vi "integer to 7-seg decoder_special.vi"(0 "Integer number":u16, 2 "Display On/Off":bool, 5 "Is negative? (F)":bool) -> (7 "7-seg digit for negative":T1)   [LabVIEW 2015]
doc: "This module is intended only to display a possible error condition 'E', entering the number 8, and turn on the g segment to indicate a minus sign. Finally, it has a complete shutdown of the display, and this state takes precedence over all others."
uses:
  controls/green 7-seg display special.ctl
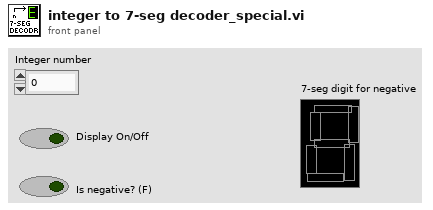
[diagram p1: front panel]
types:
  T1 = typedef "green 7-seg display special.ctl" = cluster{"a-seg":bool, "b-seg":bool, "c-seg":bool, "d-seg":bool, "e-seg":bool, "f-seg":bool, "g-seg":bool}
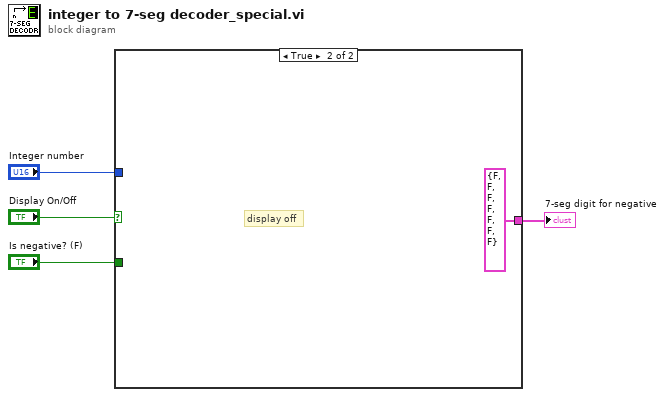
[diagram p0: block diagram]
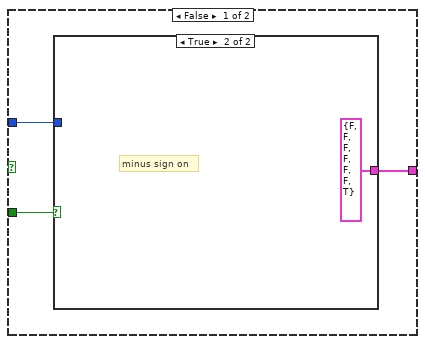
[diagram p2: hidden frame]
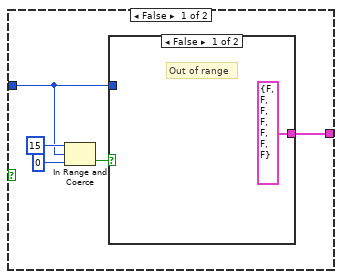
[diagram p3: hidden frame]
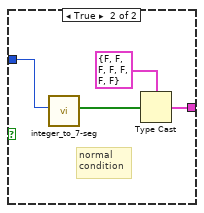
[diagram p4: hidden frame]
diagram:
  n1 = case shown="True" "Display On/Off" {
    tunnel: [w5 T1 {"a-seg"=FALSE, "b-seg"=FALSE, "c-seg"=FALSE, "d-seg"=FALSE, "e-seg"=FALSE, "f-seg"=FALSE, "g-seg"=FALSE} ("7-seg digit for negative")] -> w1
    tunnel: "Is negative? (F)" -> [w7 _]
    tunnel: "Integer number" -> [w6 _]
    frame False {
      n2 = case shown="True" w7 {
        tunnel: [w9 T1 {"a-seg"=FALSE, "b-seg"=FALSE, "c-seg"=FALSE, "d-seg"=FALSE, "e-seg"=FALSE, "f-seg"=FALSE, "g-seg"=TRUE} ("7-seg digit for negative")] -> w5
        tunnel: w6 -> [w8 _]
        frame False {
          n3 = In Range and Coerce(upper limit=u16 15, x=w8, lower limit=u16 0) -> (In Range?=w10:bool)  [unwired: 1 out]
          n4 = case shown="False" w10 {
            tunnel: w8 -> [_ w17]
            tunnel: [T1 {"a-seg"=FALSE, "b-seg"=FALSE, "c-seg"=FALSE, "d-seg"=FALSE, "e-seg"=FALSE, "f-seg"=FALSE, "g-seg"=FALSE} ("7-seg digit for negative") w15] -> w9
            frame False {
              # "Out of range"
            }
            frame True {
              # "normal \ncondition"
              n5 = call "integer_to_7-seg.vi"("Entero"=w17) -> ("7-seg"=w14:bool[])  [unwired: 10 in]
              n6 = Type Cast(type=T1 {"a-seg"=FALSE, "b-seg"=FALSE, "c-seg"=FALSE, "d-seg"=FALSE, "e-seg"=FALSE, "f-seg"=FALSE, "g-seg"=FALSE} ("7-seg digit for negative"), x=w14) -> (*(type *) &x=w15:T1)
            }
          }
        }
        frame True {
          # "minus sign on"
        }
      }
    }
    frame True {
      # "display off"
    }
  }
  "7-seg digit for negative" <- w1
